vi "Self-Test.vi"(8 "error in (no error)":errorcluster, 11 "VISA resource name":refnum<visa-resource-name>) -> (0 "error out":errorcluster, 1 "Self-Test Result Message":string, 2 "Self-Test Result Code":i32, 3 "VISA resource name out":refnum<visa-resource-name>)   [LabVIEW 2019, in "BK Precision 8500B Series.lvlib"]
doc: "Runs the instrument's self-test routine and returns the test results."
uses:
  <instrlib>/BK Precision 8500B Series/BK Precision 8500B Series.lvlib
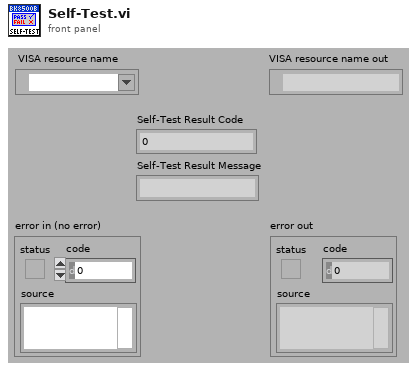
[diagram p1: front panel]
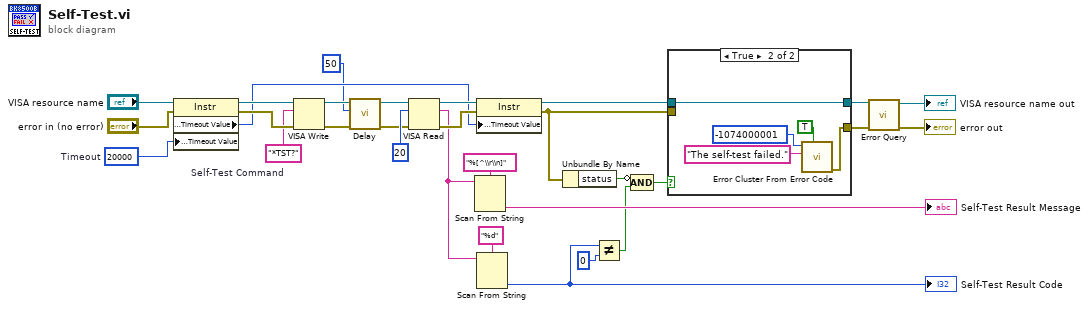
[diagram p0: block diagram]
diagram:
  w19 = u32 20000  # Timeout
  w15 = "*TST?"  # Self-Test Command
  n1 = property class="Instr"(reference="VISA resource name", error in="error in (no error)", "General Settings:Timeout Value"=w19) -> (reference out=w17:refnum<visa-resource-name>, error out=w18:errorcluster, "General Settings:Timeout Value"=w16:u32)
  n2 = VISA Write(VISA resource name=w17, write buffer=w15, error in (no error)=w18) -> (VISA resource name out=w2:refnum<visa-resource-name>, error out=w5:errorcluster)  [unwired: 1 out]
  n3 = call <instrlib>:"Delay.vi"("error in (no error)"=w5, "Delay Time (10 ms)"=50, "VISA resource name"=w2) -> ("error out"=w4:errorcluster, "VISA resource name out"=w3:refnum<visa-resource-name>)  [unwired: 7 in]
  n4 = VISA Read(VISA resource name=w3, byte count=u32 20 ("byte count (20)"), error in (no error)=w4) -> (VISA resource name out=w28:refnum<visa-resource-name>, read buffer=w23:string, error out=w27:errorcluster)  [unwired: 1 out]
  n5 = Scan From String(format string="%[^\\r\\n]" ("Format String"), input string=w23) -> (output 1=→"Self-Test Result Message":string)  [unwired: 3 in, 3 out]
  n6 = property class="Instr"(reference=w28, error in=w27, "General Settings:Timeout Value"=w16) -> (reference out=w14:refnum<visa-resource-name>, error out=w13:errorcluster)
  n7 = Scan From String(format string="%d", input string=w23) -> (output 1=w7:i32)  [unwired: 3 in, 3 out]
  "Self-Test Result Code" <- w7
  n8 = Unbundle By Name(w13) -> ("status"=w9:bool)
  n9 = Not Equal?(x=w7, y=0) -> (x != y?=w10:bool)
  n10 = Compound Arithmetic op=AND(invert w9, w10) -> (w8:bool)
  n11 = case shown="True" w8 {
    tunnel: w14 -> [w32 w37]
    tunnel: w13 -> [w31 _]
    tunnel: [w31 w33] -> w12
    tunnel: [w32 w37] -> w11
    frame False {
    }
    frame True {
      n12 = call <vilib>:"Error Cluster From Error Code.vi"("show call chain? (False)"=TRUE, "error message (\"\")"="The self-test failed." ("Source (VI Name)"), "error code (0)"=-1074000001 ("Code")) -> ("error out"=w33:errorcluster)  [unwired: 6 in]
    }
  }
  n13 = call <instrlib>:"Error Query.vi"("error in (no error)"=w12, "VISA resource name"=w11) -> ("error out"=→"error out":errorcluster, "VISA resource name out"=→"VISA resource name out":refnum<visa-resource-name>)  [unwired: 6 in, 2 out]
